vi "compass_calibrate.vi"   [LabVIEW 2012, in "Serenity_mk2.lvrbt"]
uses:
  Serenity_mk2.lvrbt
  <vilib>/NXT/Block Support/NXT_InputPort.ctl
  <vilib>/NXT/Dual Mode Library/Sound/Tone.vi
  <vilib>/NXT/Dual Mode Library/Waits/Wait_Num.vi
types:
  T1 = typedef "NXT_InputPort.ctl" = u32
  T2 = typedef "LVHSConnector.ctl" = refnum<class "BrickReference.lvclass">
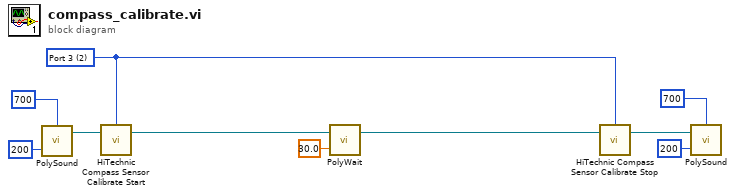
[diagram p0: block diagram]
diagram:
  w10 = T1 2 items=["Port 1", "Port 2", "Port 3", "Port 4"] ("Port")
  n1 = call-poly <vilib>:"PolySound.vi"("Duration (500 ms)"=u16 200, "Tone (440 Hz)"=u16 700) -> ("NXT/EV3"=w7:T2)  [unwired: 2 in]
  n2 = call <vilib>:"HiTechnic Compass Sensor Calibrate Start.vi"("NXT/EV3"=w7, "Port"=w10) -> ("NXT/EV3"=w9:T2)  [unwired: 2 in]
  n3 = call-poly <vilib>:"PolyWait.vi"("Time (1 sec)"=sgl 30.0, "NXT/EV3"=w9) -> ("NXT/EV3"=w8:T2)  [unwired: 2 in]
  n4 = call <vilib>:"HiTechnic Compass Sensor Calibrate Stop.vi"("NXT/EV3"=w8, "Port"=w10) -> ("NXT/EV3"=w1:T2)  [unwired: 1 in, 1 out]
  n5 = call-poly <vilib>:"PolySound.vi"("Duration (500 ms)"=u16 200, "NXT/EV3"=w1, "Tone (440 Hz)"=u16 700) -> ()  [unwired: 1 in, 1 out]
